vi "ScaleNative.vi"(5 "Scale Turn":dbl=18000.0 format="%#_13g", 7 "Scale Drive":dbl=36000.0 format="%#_13g", 9 "Left":dbl(slide) scale=1.0..-1.0, 10 "Forward":dbl(slide) scale=-1.0..1.0) -> (1 "CounterClock Scaled":dbl(slide) scale=100000.0..-100000.0, 2 "Forward Scaled":dbl(slide) scale=-100000.0..100000.0)   [LabVIEW 2017]
panel:
  # "Out (after scaling)"
  # "Input (percentage)"
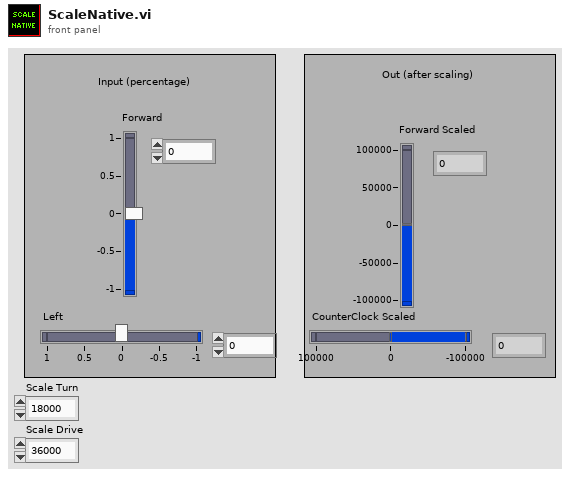
[diagram p1: front panel]
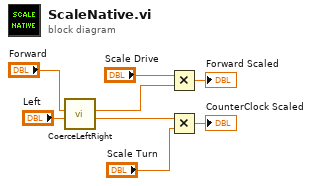
[diagram p0: block diagram]
diagram:
  n1 = call "CoerceLeftRight.vi"("Left"="Left", "Forward"="Forward") -> ("Left"=w1:dbl, "Forward"=w2:dbl)  [unwired: 8 in]
  n2 = Multiply(x="Scale Drive", y=w2) -> (x*y=→"Forward Scaled":dbl)
  n3 = Multiply(x=w1, y="Scale Turn") -> (x*y=→"CounterClock Scaled":dbl)
